vi "Add Publisher Instance Command.vi"(8 "error in":errorcluster, 10 "New Publisher":T1, 11 "CIFCorePlugin in":refnum<class "CIFCorePlugin.lvclass">) -> (0 "error out":errorcluster, 3 "CIFCorePlugin out":refnum<class "CIFCorePlugin.lvclass">)   [LabVIEW 2021, in "CIFCorePlugin.lvclass"]
uses:
  CIFCorePlugin.lvclass
  Common/Typedef/FIFO Publisher.ctl
  <vilib>/CIF Foundation/CIF Channels Core/ChannelCommon/typedef/New FIFO Instance Configuration.ctl
  CIFCorePlugin.lvclass/CIFCorePlugin.ctl
  Typedef/gRPC to Main Commands.ctl
  fc840df3-1f18-41b1-8f0e-72595bdcb8f9.vi
  <vilib>/CIF Foundation/CIF CIPC/SubVIs/Check Error.vi
  <vilib>/CIF Foundation/CIF CIPC/SubVIs/Get Element Write Position.vi
  <vilib>/CIF Foundation/CIF CIPC/SubVIs/Notify Of New Write.vi
  <vilib>/CIF Foundation/CIF CIPC/SubVIs/Get dll Path.vi
  <vilib>/CIF Foundation/CIF CIPC/SubVIs/Get Element Info Variant.vi
  <vilib>/Utility/error.llb/Trim Whitespace.vi
  <vilib>/Utility/error.llb/Error Cluster From Error Code.vi
  Typedef/gRPC to Main Command Payload.ctl
  <vilib>/CIF Foundation/CIF Channels Core/ChannelCommon/ChannelCommon.lvlib
  Common/CIFCoreCommon.lvlib
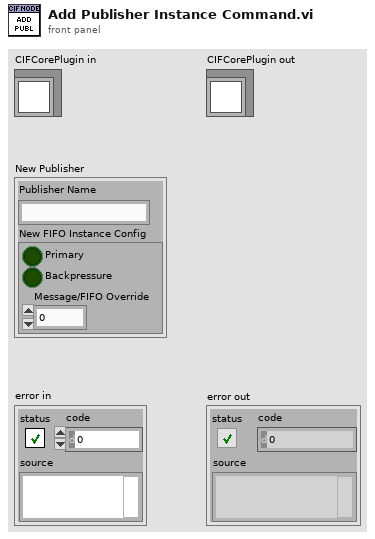
[diagram p1: front panel]
types:
  T1 = typedef "CIFCoreCommon.lvlib/FIFO Publisher.ctl" = cluster{"Publisher Name":string, "New FIFO Instance Config":T2}
  T2 = typedef "ChannelCommon.lvlib/New FIFO Instance Configuration.ctl" = cluster{"Primary":bool, "Backpressure":bool, "Message/FIFO Override":u32}
  T3 = typedef "gRPC to Main Command Payload.ctl" = cluster{"OOB_Rx Command":T4, "Array Index":i32}
  T4 = typedef "CIFCorePlugin.lvclass/gRPC to Main Commands.ctl" = enum8{"Start", "Pause", "Stop", "RefreshStats", "UpdateConfig", "Update Clock Map", "Connect Channel", "Force Channel", "Add Publisher Instance", "Remove Publisher Instance"}
  T5 = typedef "CIFCorePlugin.lvclass/gRPC to Main DVR.ctl" = refnum<data-value>
  T6 = typedef "CIFCoreCommon.lvlib/gRPC to Main Data.ctl" = cluster{"Config Data":variant, "Connections":T7[], "Forces":T8[], "Clock Conversion":T9, "Publisher Instance":T1}
  T7 = typedef "CIFCoreCommon.lvlib/Channel Connection Data.ctl" = cluster{"Publisher Name":string, "Subscriber Name":string, "Connection Data":u8[]}
  T8 = typedef "CIFCoreCommon.lvlib/Channel Force Data.ctl" = cluster{"Channel Name":string, "Force Data":u8[], "Force Active":bool}
  T9 = typedef "Time_CIF_U.lvlib/Clock Conversion Map.ctl" = map{u8, cluster{"Last Reset":i64, "Offset Pair":T10, "Slope":dbl, "1/Slope":dbl}}
  T10 = typedef "Time_CIF_U.lvlib/Timestamp Pair.ctl" = cluster{"System Time":i64, "External Time":i64}
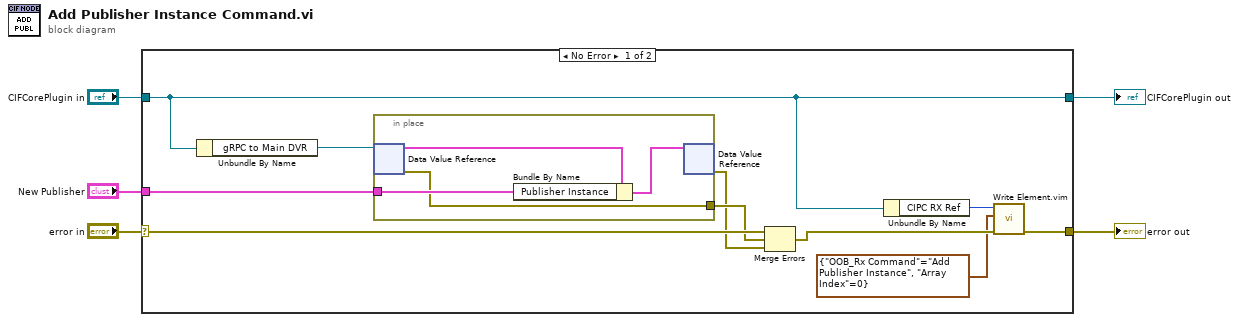
[diagram p0: block diagram]
diagram:
  n1 = case shown="No Error" "error in" {
    selector: "error in" -> [w10 w21]
    tunnel: [w15 w21] -> w4
    tunnel: "CIFCorePlugin in" -> [w13 w20]
    tunnel: [w13 w20] -> w2
    tunnel: "New Publisher" -> [w11 _]
    frame No Error {
      n2 = Unbundle By Name(w13) -> ("gRPC to Main DVR"=w12:T5)
      n3 = in-place {
        in-place-border: w11 -> [w17]
        in-place-border: [w16] -> w9
        n4 = in-place-dvr #1(w12) -> (w19:T6, w16:errorcluster)
        n5 = Bundle By Name(cluster=w19, "Publisher Instance"=w17) -> (w18:T6)
        n6 = in-place-dvr #1(w18) -> (w8:errorcluster)  [unwired: 1 out]
      }
      n7 = Merge Errors(w10, w9, w8) -> (w7:errorcluster)
      n8 = Unbundle By Name(w13) -> ("CIPC RX Ref"=w14:u64)
      n9 = call "Write Element.vim"("error in (no error)"=w7, "Data in"=T3 {"OOB_Rx Command"=enum."Add Publisher Instance", "Array Index"=0} ("gRCP to Main Command Payload"), "CIPC Reference in"=w14) -> ("error out"=w15:errorcluster)  [unwired: 5 in, 3 out]
    }
    frame Error {
    }
  }
  "error out" <- w4
  "CIFCorePlugin out" <- w2
